vi "Setmessage_a.vi"(8 "error in (no error)":errorcluster, 10 "Set_Val":T1, 11 "OneOfTemplate in":refnum<class "Greeter_req_req_oneof.lvclass">) -> (0 "error out":errorcluster, 3 "OneOfTemplate out":refnum<class "Greeter_req_req_oneof.lvclass">)   [LabVIEW 2019, in "Generated_server.lvlib" / "Greeter_req_req_oneof.lvclass"]
uses:
  Greeter_req_req_oneof.lvclass
  Greeter_MessageA.ctl
  Greeter_MessageA_oneof_a/Greeter_MessageA_oneof_a.lvclass
  Greeter_req_req_oneof.lvclass/Greeter_req_req_oneof.ctl
  Generated_server.lvlib
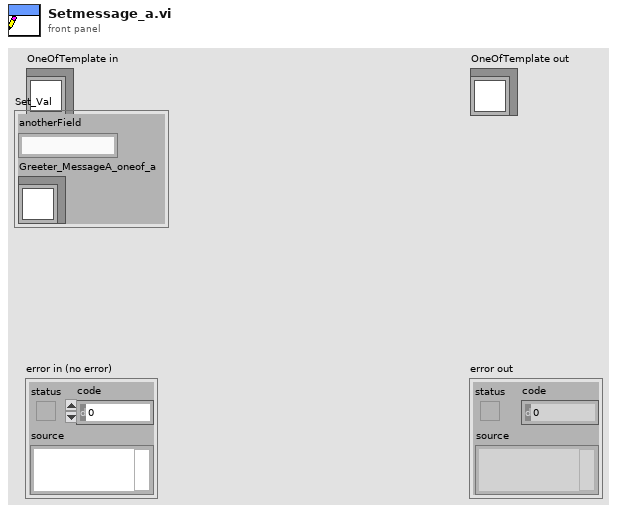
[diagram p1: front panel]
types:
  T1 = typedef "Generated_server.lvlib/Greeter_MessageA.ctl" = cluster{"anotherField":string, "Greeter_MessageA_oneof_a":refnum<class "Greeter_MessageA_oneof_a.lvclass">}
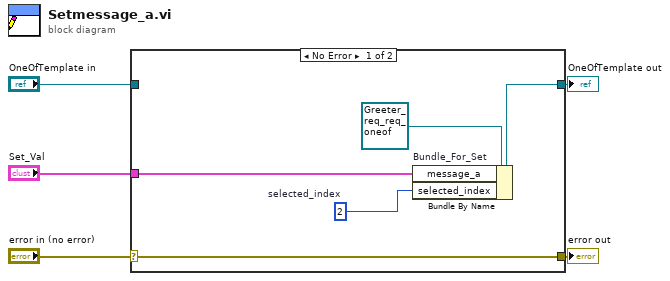
[diagram p0: block diagram]
diagram:
  n1 = case shown="No Error" "error in (no error)" {
    selector: "error in (no error)" -> [w10 w11]
    tunnel: [w10 w11] -> w4
    tunnel: [w9 w12] -> w2
    tunnel: "OneOfTemplate in" -> [_ w12]
    tunnel: "Set_Val" -> [w8 _]
    frame No Error {
      w7 = 2  # selected_index
      n2 = Bundle By Name "Bundle_For_Set"(cluster=refnum<class "Greeter_req_req_oneof.lvclass"> refnum ("OneOfTemplate in"), "message_a"=w8, "selected_index"=w7) -> (w9:refnum<class "Greeter_req_req_oneof.lvclass">)
    }
    frame Error {
    }
  }
  "error out" <- w4
  "OneOfTemplate out" <- w2
